vi "Rx Streaming (Four Channels) (Host).vi"() -> ()   [LabVIEW 2020]
doc: "This template is for the Simple NI-USRP Streaming design, a design that shows the basics of streaming data from an NI 294x/295x device. Refer to the block diagram for more information about how to use this template."
uses:
  SubVIs/Start Trigger.ctl
  <vilib>/userdefined/Silver/nirio_resource_slv.ctl
  <vilib>/Utility/error.llb/DialogType.ctl
  <vilib>/measure/maspectr.llb/FFT Power Spectrum and PSD for 1 Chan (CDB).vi
  <vilib>/measure/NI_MAPro.lvlib
panel:
  out "elements in fifo":u32[](array[numeric])
  out "error out 2":errorcluster
  out "error out":errorcluster
  in  "?":bool
  in  "phases":T1={"channel 1"=0.0, "channel 2"=0.5395, "channel 3"=0.2234, "channel 4"=0.7682}
  in  "phases 2":T1 {"channel 1" scale=0.0..1.0; "channel 2" scale=0.0..1.0; "channel 3" scale=0.0..1.0; "channel 4" scale=0.0..1.0}
  in  "cut":u32=50
  out "Done":bool=TRUE
  out "packets in buf (%)":dbl(slide)=1000.0 scale=0.0..1.0
  out "samples string buffer":string
  in  "experiment name":string="01_90_01"
  in  "packet number":u32=30
  in  "?":bool=TRUE
  out "?":dbl
  out "?":dbl(knob) scale=-90.0..90.0
  out "?":cluster{dbl[], dbl[]}(graph)
  in  "rx config":T3={"transfer mode"=enum."Finite", "sample rate"=10000000.0, "number of samples"=3000, "start trigger"=enum."Immediate", "daughterboard 0 config"={"rf enable 0"=TRUE, "rf config 0"={"antenna"="RX1", "frequency"=2475000000.0, "gain"=40.0}, "rf enable 1"=TRUE, "rf config 1"={"antenna"="RX2", "frequency"=2475000000.0, "gain"=40.0}, "lo configuration"=enum."Import"}, "daughterboard 1 config"={"rf enable 2"=TRUE, "rf config 2"={"antenna"="RX1", "frequency"=2475000000.0, "gain"=40.0}, "rf enable 3"=TRUE, "rf config 3"={"antenna"="RX2", "frequency"=2475000000.0, "gain"=40.0}, "lo configuration"=enum."Shared and Export"}} {"daughterboard 1 config"."rf config 3"."gain" format="%#.1f"; "daughterboard 1 config"."rf config 3"."frequency" format="%#.3pHz"; "daughterboard 1 config"."rf config 2"."gain" format="%#.1f"; "daughterboard 1 config"."rf config 2"."frequency" format="%#.3pHz"; "daughterboard 0 config"."rf config 1"."gain" format="%#.1f"; "daughterboard 0 config"."rf config 1"."frequency" format="%#.3pHz"; "daughterboard 0 config"."rf config 0"."gain" format="%#.1f"; "daughterboard 0 config"."rf config 0"."frequency" format="%#.3pHz"; "sample rate" format="%#.3pS/s"}
  out "acquiring":bool caption="Acquiring"
  in  "USRP RIO device":T4="RIO0" caption="USRP RIO Device"
  in  "reference frequency source":string(combo)="Internal" caption="Reference Frequency Source"
  in  "indicator tab":T5(tab)
  out "power spectrum":cluster{"f0":dbl, "df":dbl, "magnitude":dbl[]}[](graph) caption="Power Spectrum"
  out "iq data":waveform(dbl)[](graph) caption="I & Q Data"
  out "rx.coerced config":T6 caption="Coerced Configurations" {"channel 3"."sample rate" format="%#.3pS/s"; "channel 3"."gain" format="%#_1f"; "channel 3"."if2 lo" format="%#.3pHz"; "channel 3"."if1 lo" format="%#.3pHz"; "channel 3"."frequency" format="%#.3pHz"; "channel 2"."sample rate" format="%#.3pS/s"; "channel 2"."gain" format="%#_1f"; "channel 2"."if2 lo" format="%#.3pHz"; "channel 2"."if1 lo" format="%#.3pHz"; "channel 2"."frequency" format="%#.3pHz"; "channel 1"."sample rate" format="%#.3pS/s"; "channel 1"."gain" format="%#_1f"; "channel 1"."if2 lo" format="%#.3pHz"; "channel 1"."if1 lo" format="%#.3pHz"; "channel 1"."frequency" format="%#.3pHz"; "channel 0"."sample rate" format="%#.3pS/s"; "channel 0"."gain" format="%#_1f"; "channel 0"."if2 lo" format="%#.3pHz"; "channel 0"."if1 lo" format="%#.3pHz"; "channel 0"."frequency" format="%#.3pHz"}
  in  "rx.stop":bool
  # "This template shows the basics of streaming data on a USRP-2945/2955 device. Open the Project Documentation folder of the sample project and select Simple NI-USRP Streaming 2945 2955.html for information about using LO sharing with this template."
  # "Simple Rx Streaming"
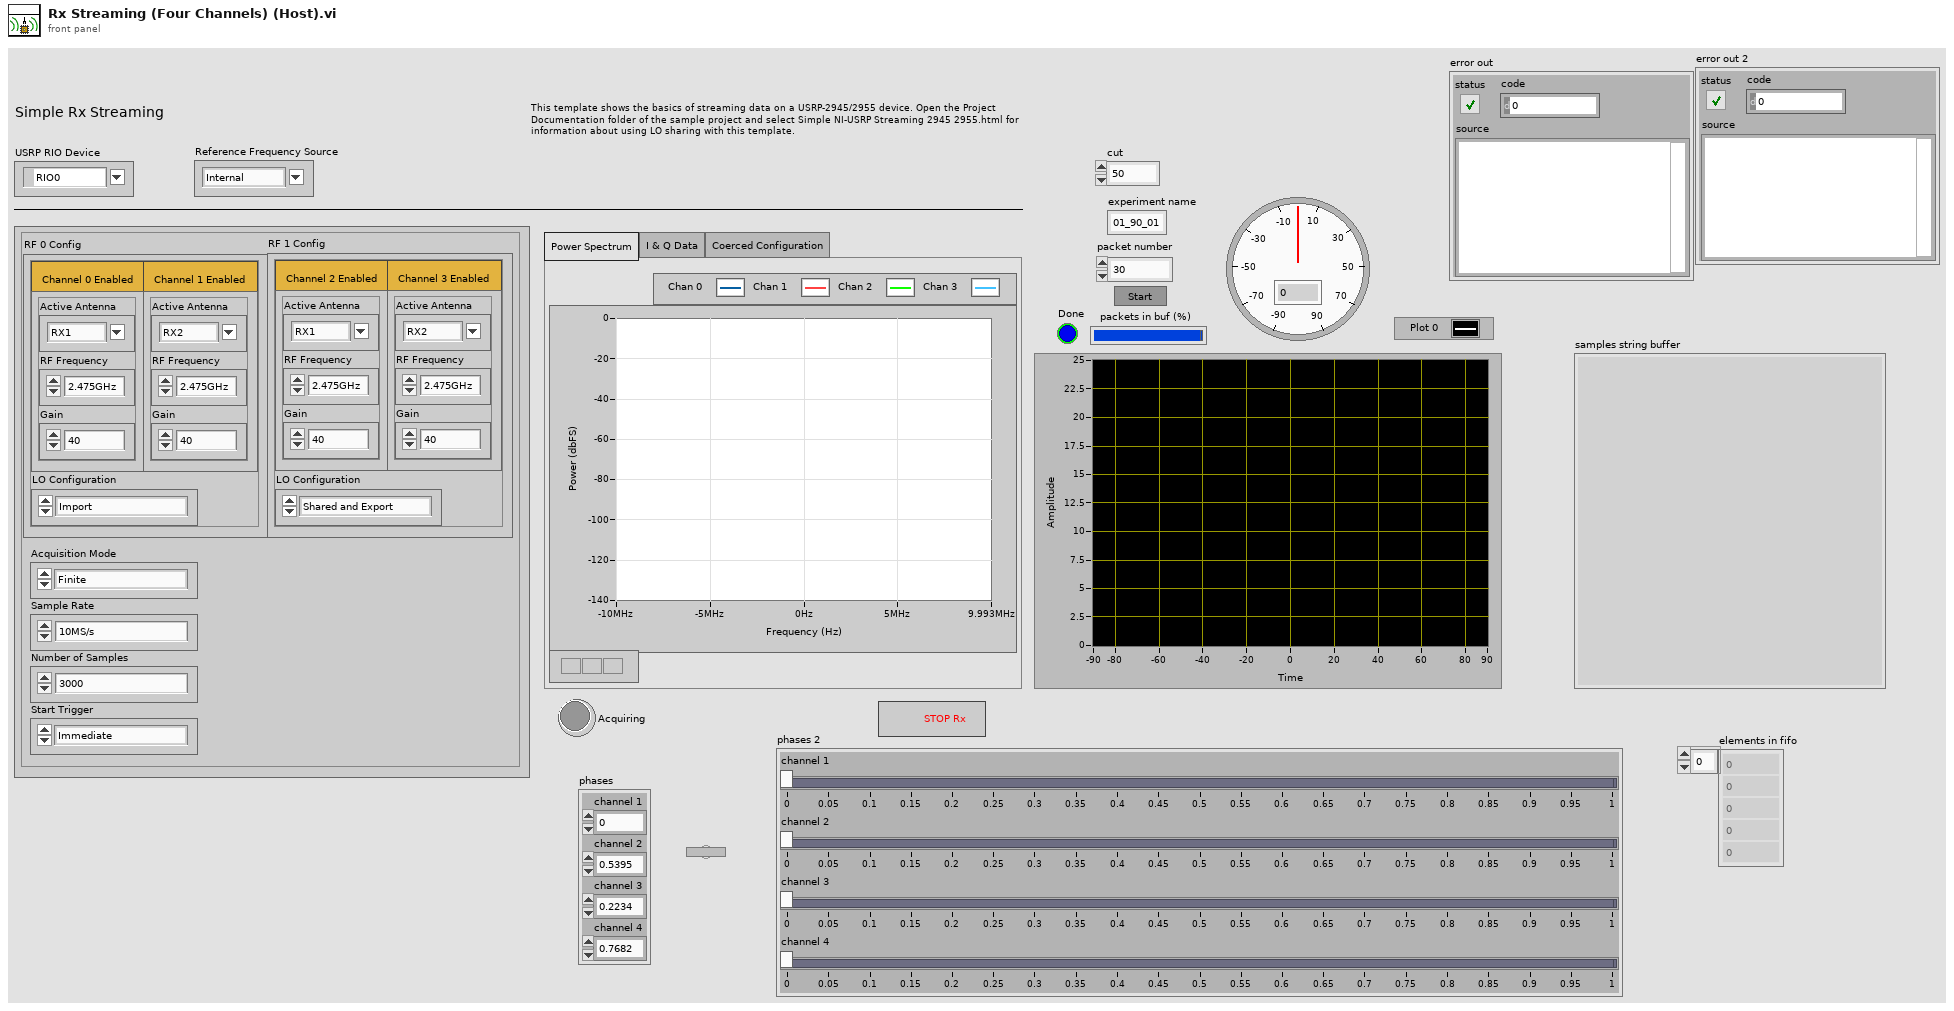
[diagram p1: front panel]
types:
  T1 = cluster{"channel 1":dbl, "channel 2":dbl, "channel 3":dbl, "channel 4":dbl}
  T2 = typedef "Start Trigger.ctl" = enum8{"Software", "Digital Edge", "Rx Start Trigger", "Tx Start Trigger", "Immediate", "Future Time Event"}
  T3 = cluster{"transfer mode":enum16{"Finite", "Continuous"}, "sample rate":dbl, "number of samples":u32, "start trigger":T2, "daughterboard 0 config":cluster{"rf enable 0":bool, "rf config 0":cluster{"antenna":string, "frequency":dbl, "gain":dbl}, "rf enable 1":bool, "rf config 1":cluster{"antenna":string, "frequency":dbl, "gain":dbl}, "lo configuration":enum16{"Independent", "Import", "Shared and Export", "Reimport", "Shared"}}, "daughterboard 1 config":cluster{"rf enable 2":bool, "rf config 2":cluster{"antenna":string, "frequency":dbl, "gain":dbl}, "rf enable 3":bool, "rf config 3":cluster{"antenna":string, "frequency":dbl, "gain":dbl}, "lo configuration":enum16{"Independent", "Import", "Shared and Export", "Reimport", "Shared"}}}
  T4 = typedef "nirio_resource_slv.ctl" = tag
  T5 = enum32{"Power Spectrum", "I & Q Data", "Coerced Configuration"}
  T6 = cluster{"channel 0":cluster{"frequency":dbl, "if1 lo":dbl, "if2 lo":dbl, "gain":dbl, "sample rate":dbl}[], "channel 1":cluster{"frequency":dbl, "if1 lo":dbl, "if2 lo":dbl, "gain":dbl, "sample rate":dbl}[], "channel 2":cluster{"frequency":dbl, "if1 lo":dbl, "if2 lo":dbl, "gain":dbl, "sample rate":dbl}[], "channel 3":cluster{"frequency":dbl, "if1 lo":dbl, "if2 lo":dbl, "gain":dbl, "sample rate":dbl}[], "device id":i32}
  T7 = typedef "DialogType.ctl" = u16
  T8 = typedef "Rx Channels.ctl" = cluster{"rx config":cluster{"channel configuration":cluster{"channel enable":bool, "channel configuration":cluster{"antenna":string, "frequency":dbl, "lo frequency":dbl, "level":dbl}}[], "transfer mode":enum16{"Finite", "Continuous"}, "sample rate":dbl, "number of samples":u32, "start trigger":T2}, "reference frequency source":string, "rx.data sink":enum16{"SFP Port 0", "SFP Port 1", "Host"}, "rx.enabled channels":string[], "vertical range":dbl[], "rx.coerced configurations":cluster{"coerced frequencies":dbl[], "coerced lo frequencies":dbl[], "coerced levels":dbl[], "coerced sample rates":dbl[]}}
  T9 = typedef "niUsrpRio Config v1 Host.lvlib/niUsrpRio Session.ctl" = cluster{"FPGA Interface":refnum<k20>, "RIO Interface Number":u32, "Data Clock Rate":u32, "FPGA Data Clock Rate":u32, "Global Settings Register Bus":T10, "Radio 0 Settings Register Bus":T10, "Radio 1 Settings Register Bus":T10, "Radio Settings Bus Semaphore":T11, "DB Queues":T12[], "Characterization Data Valid?":bool, "EEPROM Header":T13, "Device Data Header":T14, "EEPROM Characterization Header":T15, "Characterization Data":T16[], "FPGA Current Version":u32, "FPGA Oldest Compatible Version":u32, "Fixed Logic Current Version":u32, "Fixed Logic Oldest Compatible Version":u32, "FPGA Radio Settings Bus Current Version":u32, "FPGA Radio Settings Bus Oldest Compatible Version":u32, "FPGA Board Config Current Version":u32, "FPGA Board Config Oldest Compatible Version":u32, "Daughterboard Clock Rate":u32, "daughterboard configuration session handles":u64[]}
  T10 = typedef "niInstr Register Bus v0 Host.lvlib/Register Bus Session.ctl" = refnum<queue>
  T11 = typedef "Semaphore RefNum" = refnum<k1>
  T12 = typedef "niUsrpRio Config v1 Host.lvlib/DB Queue Reference.ctl" = refnum<queue>
  T13 = typedef "niUsrpRio Config v1 Host.lvlib/EEPROM Header.ctl" = cluster{"Checksum":u32, "Product Code":u16, "Hardware Current Version":u16, "Hardware Oldest Compatible Version":u16, "EEPROM Map Current Version":u16, "EEPROM Map Oldest Compatible Version":u16, "User Password":string, "Pointer to Factory Header":u32, "Pointer to User Header":u32, "Recommended Interval":u16, "Number of Reserved Bytes":i32, "Number of Daughterboards":u8, "Daughterboard IDs":u16[], "Daughterboard Serial Numbers":string[]}
  T14 = typedef "niUsrpRio Config v1 Host.lvlib/EEPROM Device Data Header.ctl" = cluster{"Checksum":u32, "Number of Channels":u8, "Number of Gain Settings":u16[], "Pointer to Characterization Data":u32[], "Number of Reserved Bytes":i32, "Number of Frequencies":u16[]}
  T15 = typedef "niUsrpRio Config v1 Host.lvlib/EEPROM Characterization Header.ctl" = cluster{"Checksum":u32, "Date":timestamp, "Temperature":sgl, "Misc. Info":string, "Pointer to Device Data Header":u32, "Number of Reserved Bytes":i32}
  T16 = typedef "niUsrpRio Config v1 Host.lvlib/Characterization Data.ctl" = cluster{"Gains[dB]":dbl[], "Frequencies [Hz]":dbl[], "IQ Imbalance Table":T17[], "Measured Gains[dB]":dbl[][]}
  T17 = typedef "niUsrpRio Config v1 Host.lvlib/IQ Imbalance.ctl" = cluster{"Gain Imbalance [linear]":dbl, "Phase Imbalance [radians]":dbl, "Offset":cdb}
  T18 = cluster{"coerced frequencies":dbl[], "coerced if1 frequencies":dbl[], "coerced if2 frequencies":dbl[], "coerced gain":dbl[], "coerced sample rates":dbl[]}
  T19 = cluster{"frequency":dbl, "if1 lo":dbl, "if2 lo":dbl, "gain":dbl, "sample rate":dbl}[]
  T20 = cluster{"frequency":dbl, "if1 lo":dbl, "if2 lo":dbl, "gain":dbl, "sample rate":dbl}
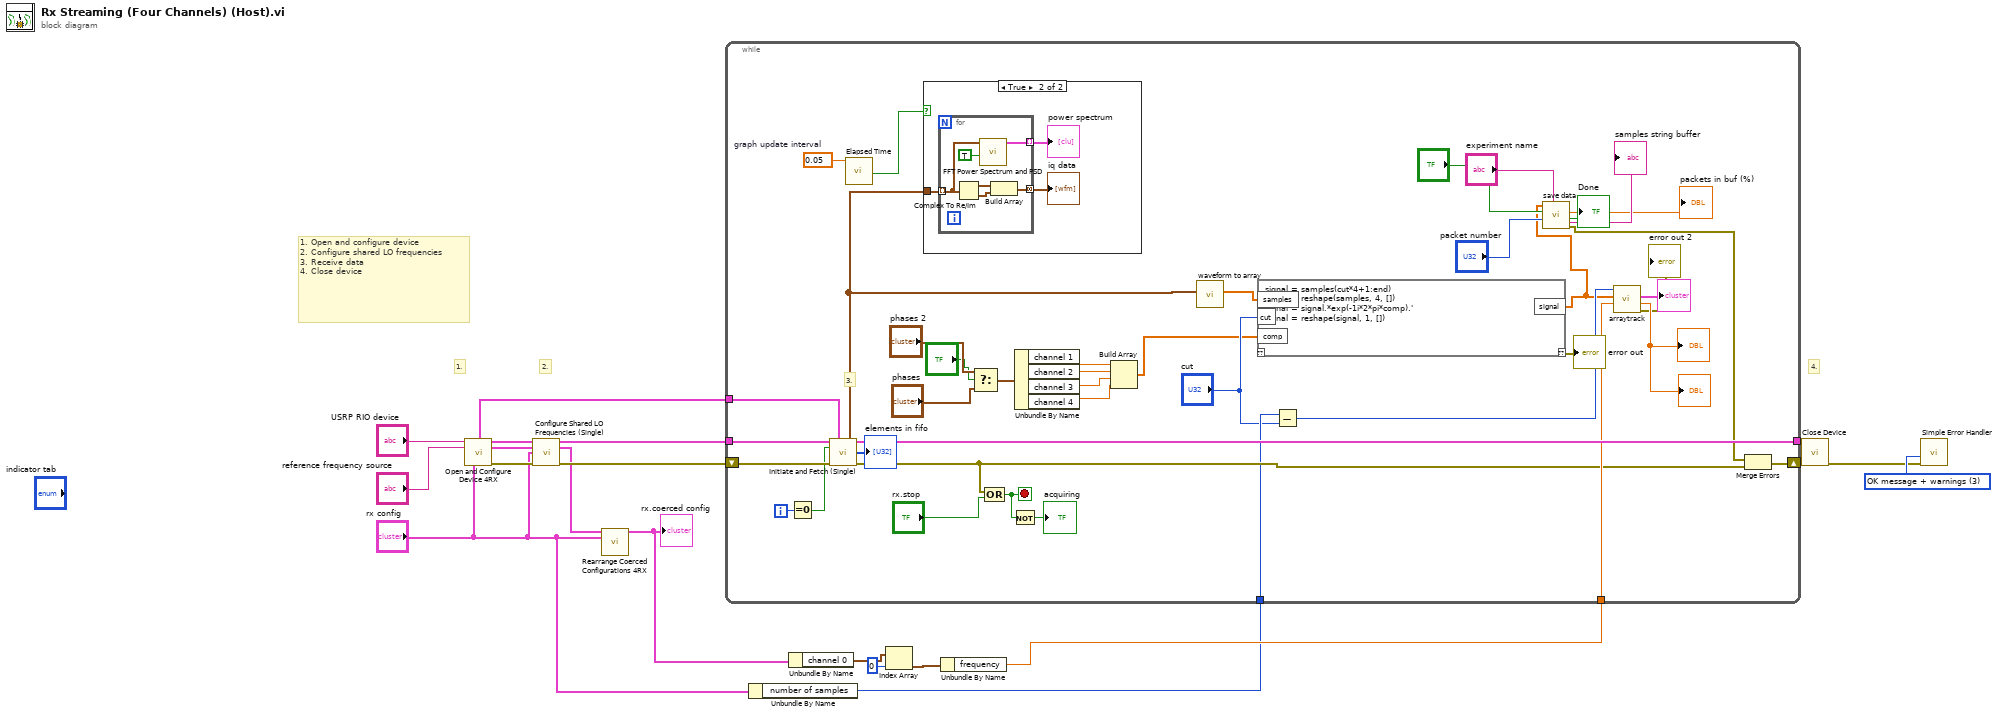
[diagram p0: block diagram]
diagram:
  w20 = T7 3 items=["no dialog", "OK message", "continue or stop message", "OK message + warnings", "continue/stop + warnings"] ("type of dialog (OK msg:1)")
  # "2."
  # "4."
  # "1. Open and configure device\n2. Configure shared LO frequencies\n3. Receive data\n4. Close device"
  # "1."
  n1 = call "Open and Configure Device 4RX.vi"("USRP RIO Device"="USRP RIO device", "reference frequency source"="reference frequency source", "rx config"="rx config") -> ("rx channels"=w14:T8, "niUsrpRio Session (out)"=w13:T9, "rx.coerced configurations"=w9:T18, "error out"=w10:errorcluster)  [unwired: 9 in]
  n2 = call "Configure Shared LO Frequencies (Single).vi"("niUsrpRio Session"=w13, "rx.coerced config"=w9, "rx config"="rx config", "error in"=w10) -> ("niUsrpRio Session (out)"=w12:T9, "rx.coerced config out"=w8:T18, "error out"=w11:errorcluster)  [unwired: 9 in]
  n3 = call "Rearrange Coerced Configurations 4RX.vi"("rx.coerced configurations"=w8, "rx config"="rx config") -> ("coerced configurations"=w7:T6)  [unwired: 13 in]
  "rx.coerced config" <- w7
  n4 = Unbundle By Name("rx config") -> ("number of samples"=w1:u32)
  n5 = Unbundle By Name(w7) -> ("channel 0"=w5:T19)
  n6 = Index Array(array=w5, index=0) -> (element=w6:T20)
  n7 = Unbundle By Name(w6) -> ("frequency"=w3:dbl)
  n8 = while {
    tunnel: w12 -> [w59]
    tunnel: [w57] -> w15
    tunnel: w14 -> [w54]
    shift-right: [w38] -> w16
    shift-left: w11 -> [w60]
    tunnel: w3 -> [w48]
    tunnel: w1 -> [w37]
    i -> [w58]
    stop <- w55 stop-if-true
    w52 = 0.05  # graph update interval
    # "3."
    # "Acquire and Fetch a waveform"
    n9 = Equal To 0?(x=w58) -> (x = 0?=w51:bool)
    n10 = call "Initiate and Fetch (Single).vi"("niUsrpRio Session"=w59, "rx channels"=w54, "first iteration"=w51, "error in"=w60) -> ("niUsrpRio Session (out)"=w57:T9, "complex baseband data"=w49:waveform(cdb)[], "elements in fifo"=→"elements in fifo":u32[], "error out"=w39:errorcluster)  [unwired: 8 in]
    n11 = call "Elapsed Time"("Time Target (s)"=w52) -> ("Time has Elapsed"=w53:bool)  [unwired: 11 in, 7 out]
    n12 = case shown="True" w53 {
      tunnel: w49 -> [_ w64]
      frame False {
      }
      frame True {
        n13 = for {
          tunnel: [w68] -> w63 mode=concatenating
          tunnel: [w66] -> w62 mode=indexing
          tunnel: w64 -> [w67] mode=indexing
          n14 = Complex To Re/Im(x + iy=w67) -> (x=w70:waveform(dbl), y=w69:waveform(dbl))
          n15 = call-poly <vilib>:"FFT Power Spectrum and PSD.vi"("dB On (F)"=TRUE, "time signal"=w67) -> ("Power Spectrum / PSD"=w66:cluster{"f0":dbl, "df":dbl, "magnitude":dbl[]})  [unwired: 6 in, 3 out]
          n16 = Build Array(w70, w69) -> (w68:waveform(dbl)[])
        }
        "power spectrum" <- w62
        "iq data" <- w63
      }
    }
    n17 = Select(t="phases 2", s="?", f="phases") -> (s? t:f=w34:T1)
    n18 = Compound Arithmetic op=OR(w39, "rx.stop") -> (w55:bool)
    n19 = Not(x=w55) -> (.not. x?=→"acquiring":bool)
    n20 = Unbundle By Name(w34) -> ("channel 1"=w27:dbl, "channel 2"=w28:dbl, "channel 3"=w29:dbl, "channel 4"=w30:dbl)
    n21 = Build Array(w27, w28, w29, w30) -> (w26:dbl[])
    n22 = call "waveform to array.vi"("complex baseband data"=w49) -> ("Y"=w22:cdb[])  [unwired: 10 in]
    n23 = script code="signal = samples(cut*4+1:end)\nsignal = reshape(samples, 4, [])\nsignal = signal.*exp(-1i*2*pi*comp).'\nsignal = reshape(signal, 1, [])" ("Script Node")("samples"=w22, "cut"="cut", "comp"=w26) -> ("??"=→"error out":errorcluster, "signal"=w23:cdb[])  [unwired: 1 in]
    n24 = Subtract(x=w37, y="cut") -> (x-y=w36:u32)
    n25 = call "save data.vi"("experiment name"="experiment name", "packet number"="packet number", 10:"?", "samples"=w23) -> ("error out"=w41:errorcluster, "Done"=→"Done":bool, "packets in buf (%)"=→"packets in buf (%)":dbl, "samples string buffer"=→"samples string buffer":string)  [unwired: 3 in, 1 out]
    n26 = call "arraytrack.vi"("freq"=w48, "samples"=w23, "samples num"=w36) -> ("error out"=→"error out 2":errorcluster, "max"=→"?" →"?":dbl, "spectrum"=→"?":cluster{dbl[], dbl[]})  [unwired: 6 in]
    n27 = Merge Errors(w41, w39) -> (w38:errorcluster)
  }
  n28 = call "Close Device.vi"("niUsrpRio Session"=w15, "error in"=w16) -> ("error out"=w19:errorcluster)  [unwired: 13 in]
  n29 = call <vilib>:"Simple Error Handler.vi"("type of dialog (OK msg:1)"=w20, "error in (no error)"=w19) -> ()  [unwired: 3 in, 5 out]
